vi "MGCC_PlannedISD_main.vi"() -> ()   [LabVIEW 2016]
doc: "-----------------------------------------------------------------------------------------------------------------------\nCopyright <2019> <The University of Tennessee at Knoxville and the University of Tennessee Research Foundation>\nThis software is released under BSD-3 \nhttps://opensource.org/licenses/BSD-3-Clause \nAdditional license options available at https://utrf.tennessee.edu/industry/sample-agreements/\n-----------------------------------------------------------------------------------------------------------------------"
uses:
  Finite State Machine/Sub-VIs/MGCC_FntStaMach_gobal.vi
  Communication/Global communication.vi
  Model Management/Global_MdlMgmt.vi
  Communication/Global communication output.vi
  <vilib>/imath/engines/lvmath2/RunTimeEngine/Managers/WorkSpace/UID Generator.vi
  <vilib>/imath/engines/lvmath2/RunTimeEngine/BuiltInFunctions/size/NIMS_I32=size(GM,I32).vi
  <instcachedir>/0/NIMS_I32=size(GM,I32)_122058B1B3294FAEA5DC209B92B394E4.lvgen/NIMS_I32=size(GM,I32)_122058B1B3294FAEA5DC209B92B394E4_004.vi
  <vilib>/imathl/engines/lvmath/Functions/Error Handling/Create Error.vi
  <vilib>/imath/engines/lvmath2/RunTimeEngine/CommandStatement/MC_CommandStatement_break.vi
  <vilib>/imath/engines/lvmath2/RunTimeEngine/IndexRead/NIMS M(S,S).vi
  <instcachedir>/0/NIMS M(S,S)_AC51E74150A542F7991B9634C66F3096.lvgen/NIMS M(S,S)_AC51E74150A542F7991B9634C66F3096_000.vi
  <vilib>/imath/engines/lvmath2/RunTimeEngine/IndexReplace/NIMS M(S,$)=M.vi
  <instcachedir>/0/NIMS M(S,$)=M_47BFD2E070824516B94BE47F5466D205.lvgen/NIMS M(S,$)=M_47BFD2E070824516B94BE47F5466D205_000.vi
  <vilib>/imath/engines/lvmath2/RunTimeEngine/CommandStatement/NIMS_CommandStatement_MaskErr.vi
  <vilib>/imath/engines/lvmath2/RunTimeEngine/RangeToken/NIMS_Range_R2 - Integer.vi
  <instcachedir>/0/NIMS_Range_R2 - Integer_89B873E74E6E489885E44F751DD9C6BF.lvgen/NIMS_Range_R2 - Integer_89B873E74E6E489885E44F751DD9C6BF_000.vi
  <vilib>/imath/engines/lvmath2/RunTimeEngine/IndexRead/NIMS V(S).vi
  <instcachedir>/0/NIMS V(S)_0488751826AF41519A22953C041130DC.lvgen/NIMS V(S)_0488751826AF41519A22953C041130DC_000.vi
  <vilib>/imath/engines/lvmath2/RunTimeEngine/RunTimeType/NIMS_RunTimeType_From StrictType (excl LVString).vi
  <instcachedir>/0/NIMS_RunTimeType_From StrictType (excl LVString)_BBF44FB49F834B71AF7A14CCEDF8BECD.lvgen/NIMS_RunTimeType_From StrictType (excl LVString)_BBF44FB49F834B71AF7A14CCEDF8BECD_000.vi
  <vilib>/imath/engines/lvmath2/RunTimeEngine/LocalVariableDefStatement/MC_LocalVariableDefStatement_Display.vi
  <vilib>/imath/engines/lvmath2/RunTimeEngine/Managers/SymbolTable/Clear UID.vi
  <vilib>/imath/engines/lvmath2/RunTimeEngine/NodeEndStatement/NIMS_NodeEndStatement_Output.vi
  <instcachedir>/0/NIMS_NodeEndStatement_Output_53EC0D466D134D7ABD903AC30B43404B.lvgen/NIMS_NodeEndStatement_Output_53EC0D466D134D7ABD903AC30B43404B_001.vi
  <instcachedir>/0/NIMS_NodeEndStatement_Output_53EC0D466D134D7ABD903AC30B43404B.lvgen/NIMS_NodeEndStatement_Output_53EC0D466D134D7ABD903AC30B43404B_011.vi
  <vilib>/imath/engines/lvmath2/RunTimeEngine/ErrorHandling/NIMS_Finalize Error.vi
  <vilib>/imath/engines/lvmath2/RunTimeEngine/BuiltInFunctions/abs/NIMS_abs(signed).vi
  <instcachedir>/0/NIMS_abs(signed)_C4FCB8E6058B49B797C7C8D53CA5F6EC.lvgen/NIMS_abs(signed)_C4FCB8E6058B49B797C7C8D53CA5F6EC_000.vi
  <vilib>/imath/engines/lvmath2/RunTimeEngine/RunTimeType/NIMS_RunTimeType_Set Source Original Bool.vi
  <instcachedir>/0/NIMS_NodeEndStatement_Output_53EC0D466D134D7ABD903AC30B43404B.lvgen/NIMS_NodeEndStatement_Output_53EC0D466D134D7ABD903AC30B43404B_015.vi
  <vilib>/imath/engines/lvmath2/RunTimeEngine/Managers/SymbolTable/NIMS_WorkSpace.lvlib
panel:
  out "error out":errorcluster
  out "To Topology Identification":dbl[][](array[numeric])
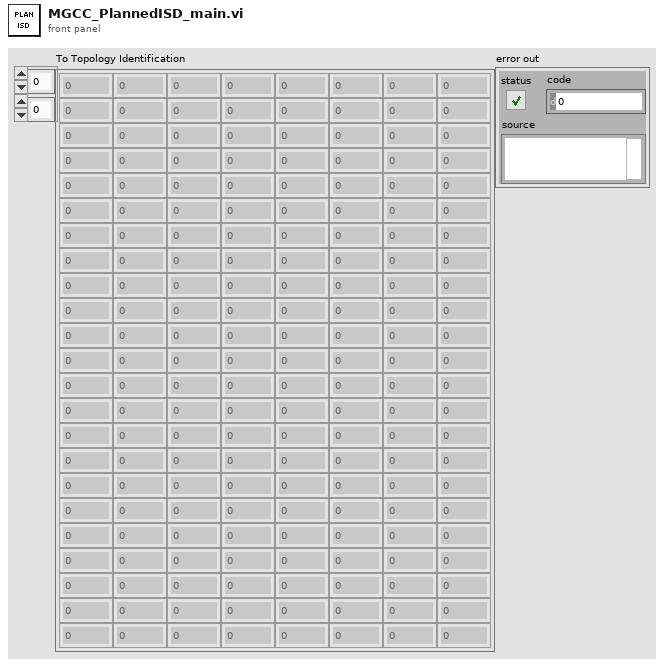
[diagram p1: front panel]
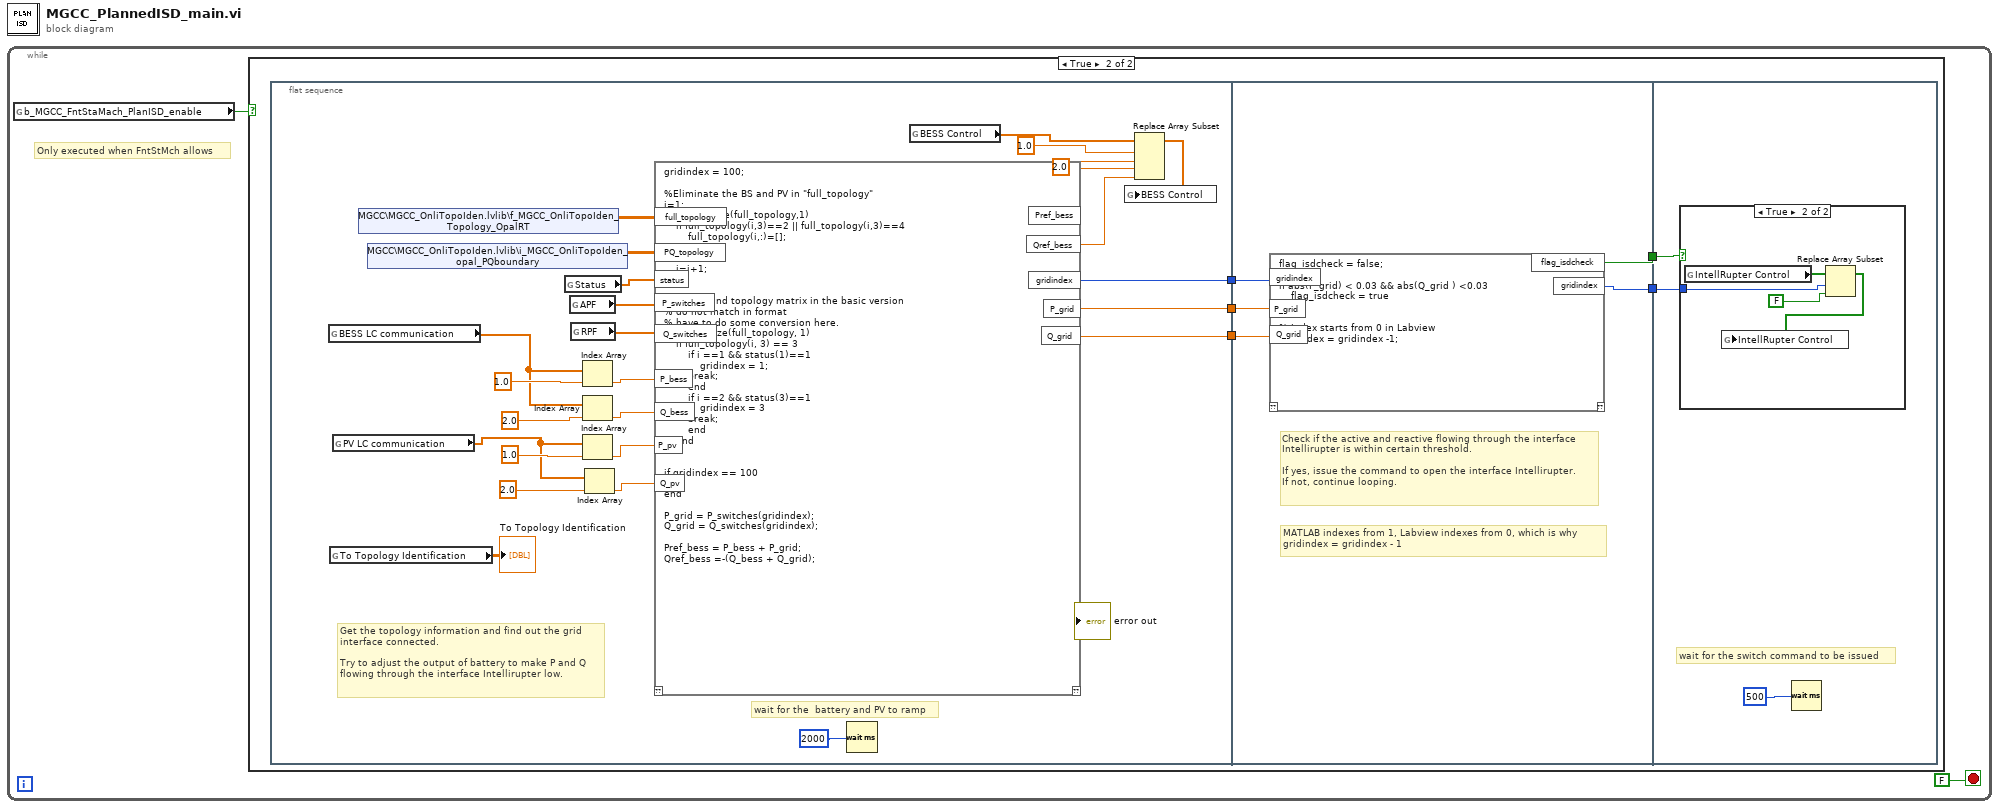
[diagram p0: block diagram]
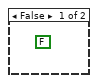
[diagram p2: hidden frame]
diagram:
  n1 = while {
    stop <- FALSE stop-if-true
    # "Only executed when FntStMch allows"
    n2 = global read "MGCC_FntStaMach_gobal.vi" "b_MGCC_FntStaMach_PlanISD_enable"() -> (w2:bool)
    n3 = case shown="True" w2 {
      frame False {
        (unwired) FALSE ("flag_isdcheck")
      }
      frame True {
        n4 = flat-sequence {
          tunnel: [w14] -> w7
          tunnel: [w13] -> w6
          tunnel: [w12] -> w5
          tunnel: w7 -> [w522]
          tunnel: w6 -> [w521]
          tunnel: w5 -> [w520]
          tunnel: [w519] -> w4
          tunnel: [w518] -> w3
          tunnel: w4 -> [w602]
          tunnel: w3 -> [w604]
          frame #0 {
            # "Get the topology information and find out the grid\ninterface connected. \n\nTry to adjust the output of battery to make P and Q\nflowing through the interface Intellirupter low."
            # "wait for the  battery and PV to ramp"
            n5 = global read "Global communication.vi" "BESS LC communication"() -> (w27:dbl[])
            n6 = global read "Global_MdlMgmt.vi" "To Topology Identification"() -> (→"To Topology Identification":dbl[][])
            n7 = global read "Global communication.vi" "PV LC communication"() -> (w22:dbl[])
            n8 = shared-variable "MGCC\\MGCC_OnliTopoIden.lvlib\\f_MGCC_OnliTopoIden_Topology_OpalRT"() -> (w33:dbl[][])  [unwired: 1 in, 1 out]
            n9 = shared-variable "MGCC\\MGCC_OnliTopoIden.lvlib\\i_MGCC_OnliTopoIden_opal_PQboundary"() -> (w32:dbl[][])  [unwired: 1 in, 1 out]
            n10 = global read "Global communication.vi" "Status"() -> (w9:dbl[])
            n11 = global read "Global communication.vi" "APF"() -> (w31:dbl[])
            n12 = global read "Global communication.vi" "RPF"() -> (w30:dbl[])
            n13 = Index Array(array=w27, index=1.0) -> (element=w25:dbl)
            n14 = Index Array(array=w27, index=2.0) -> (element=w26:dbl)
            n15 = Index Array(array=w22, index=1.0) -> (element=w21:dbl)
            n16 = Index Array(array=w22, index=2.0) -> (element=w20:dbl)
            n17 = mathscript code="gridindex = 100;\n\n%Eliminate the BS and PV in \"full_topology\"\ni=1;\nwhile i<=size(full_topology,1)\n    if full_topology(i,3)==2 || full_topology(i,3)==4\n        full_topology(i,:)=[];\n        i=i-1;\n    end\n    i=i+1;\nend\n\n% Status and topology matrix in the basic version\n% do not match in format\n% have to do some conversion here.\nfor i= 1 : size(full_topology, 1)\n    if full_topology(i, 3) == 3\n        if i ==1 && status(1)==1\n            gridindex = 1;\n        break;\n        end\n        if i ==2 && status(3)==1\n            gridindex = 3\n        break;\n        end\n    end\nend\n\nif gridindex == 100\n    \nend\n\nP_grid = P_switches(gridindex);\nQ_grid = Q_switches(gridindex);\n\nPref_bess = P_bess + P_grid;\nQref_bess =-(Q_bess + Q_grid);"("full_topology"=w33, "PQ_topology"=w32, "P_switches"=w31, "Q_switches"=w30, "P_bess"=w25, "Q_bess"=w26, "P_pv"=w21, "Q_pv"=w20, "status"=w9) -> ("??"=→"error out":errorcluster, "Pref_bess"=w10:dbl, "Qref_bess"=w8:dbl, "gridindex"=w14:i32, "P_grid"=w13:dbl, "Q_grid"=w12:dbl)  [unwired: 1 in]
            n18 = Wait (ms)(milliseconds to wait=2000) -> ()  [unwired: 1 out]
            n19 = global read "Global communication output.vi" "BESS Control"() -> (w18:dbl[])
            n20 = Replace Array Subset(array=w18, new element #1=w10, index #1=1.0, new element #2=w8, index #2=2.0) -> (w19:dbl[])
            n21 = global write "Global communication output.vi" "BESS Control"(w19) -> ()
          }
          frame #1 {
            # "MATLAB indexes from 1, Labview indexes from 0, which is why\ngridindex = gridindex - 1"
            # "Check if the active and reactive flowing through the interface\nIntellirupter is within certain threshold.\n\nIf yes, issue the command to open the interface Intellirupter.\nIf not, continue looping."
            n22 = mathscript code="flag_isdcheck = false;\n\nif abs(P_grid) < 0.03 && abs(Q_grid ) <0.03\n    flag_isdcheck = true\nend\n\n% Index starts from 0 in Labview\ngridindex = gridindex -1;"("gridindex"=w522, "P_grid"=w521, "Q_grid"=w520) -> ("flag_isdcheck"=w519:bool, "gridindex"=w518:i32)  [unwired: 1 in, 1 out]
          }
          frame #2 {
            # "wait for the switch command to be issued"
            n23 = case shown="True" w602 {
              tunnel: w604 -> [_ w607]
              frame False {
              }
              frame True {
                n24 = global read "Global communication output.vi" "IntellRupter Control"() -> (w608:bool[])
                n25 = Replace Array Subset(array=w608, new element=FALSE ("new element/subarray"), index=w607) -> (w605:bool[])
                n26 = global write "Global communication output.vi" "IntellRupter Control"(w605) -> ()
              }
            }
            n27 = Wait (ms)(milliseconds to wait=500) -> ()  [unwired: 1 out]
          }
        }
      }
    }
  }
